vi "FindRobotByRole.vi"(8 "error in (no error)":errorcluster, 9 "role":T1=enum."DefenderArea", 10 "RobotRef":refnum<class "Robot.lvclass">[](array[class]), 11 "Utilities in":refnum<class "Utilities.lvclass">) -> (0 "error out":errorcluster, 2 "Robots":refnum<class "Robot.lvclass">[](array[class]), 3 "Utilities out":refnum<class "Utilities.lvclass">)   [LabVIEW 2023, in "Utilities.lvclass"]
uses:
  Utilities.lvclass
  Robot_class/Robot.lvclass
  Robot_class/roles.ctl
  Robot_class/Robot.lvclass/Robot.ctl
  Robot_class/Read role.vi
panel:
  out "Roles":T1[](array[typedef])
  out "role 2":i32
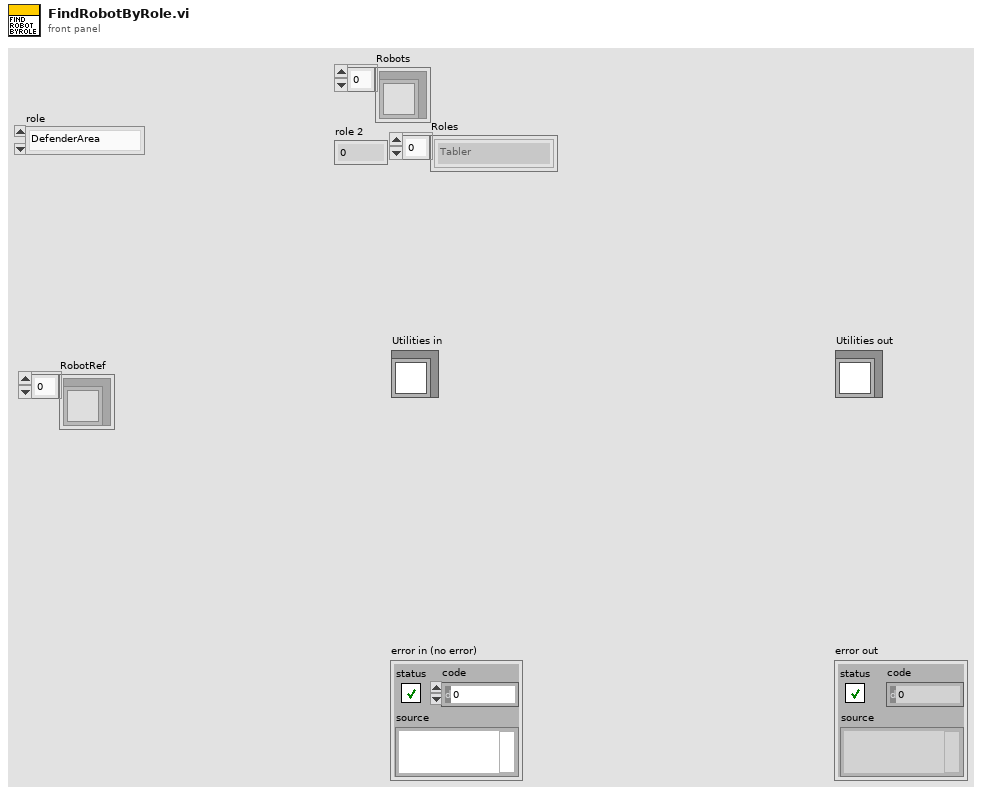
[diagram p1: front panel]
types:
  T1 = typedef "roles.ctl" = enum16{"BallChallengerAttackerVSS", "NormalAttackerVSS", "AttackerAimGoalVSS", "DefenderAreaVSS", "KeeperVSS", "Tabler", "TableFinalizer", "PrepareRollToPassRoller", "PrepareRollToPassReceiver", "SimplePassRoll", "SimplePassRollReceiver", "PenaltyDefense", "PreparePassReceiver 2", "PreparePassReceiver 1", "PassObserver", "Timeout", "Goto", "ZigZag", "None", "BallOutOfField", "DefenderArea", "Duelist", "AttackerStop", "FollowAttacker", "KeeperRole", "KickPenalty", "AttackerAimGoal", "AttackerBlock", "Marker", "Halt", "Shoot", "PassKicker", "PassReceiver", "TestRole", "PenaltyAttacker"}
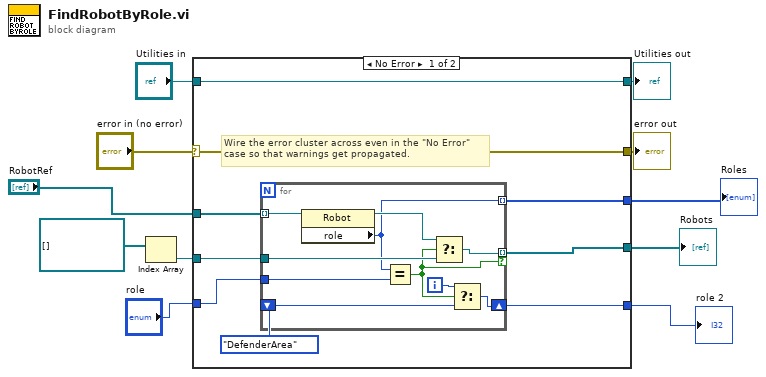
[diagram p0: block diagram]
diagram:
  n1 = Index Array(array=refnum<class "Robot.lvclass">[] []) -> (element=w6:refnum<class "Robot.lvclass">)  [unwired: 1 in]
  n2 = case shown="No Error" "error in (no error)" {
    selector: "error in (no error)" -> [w19 w32]
    tunnel: [w19 w32] -> w10
    tunnel: [w20 w31] -> w8
    tunnel: "Utilities in" -> [w20 w31]
    tunnel: [w18 _] -> w2
    tunnel: w6 -> [w14 _]
    tunnel: "RobotRef" -> [w17 _]
    tunnel: "role" -> [w16 _]
    tunnel: [w13 _] -> w3
    tunnel: [w12 _] -> w1
    frame No Error {
      # "Wire the error cluster across even in the \"No Error\"\ncase so that warnings get propagated."
      n3 = for {
        tunnel: w17 -> [w30] mode=indexing
        tunnel: w16 -> [w29]
        shift-right: [w26] -> w18
        shift-left: roles."DefenderArea" ("role") -> [w25]
        tunnel: w14 -> [w24]
        tunnel: [w23] -> w13 mode=indexing if=w22
        tunnel: [w21] -> w12 mode=indexing
        i -> [w27]
        n4 = property class="Robot"(reference=w30) -> (reference out=w28:refnum<class "Robot.lvclass">, "role"=w21:T1)  [unwired: 1 in, 1 out]
        n5 = Equal?(x=w21, y=w29) -> (x = y?=w22:bool)
        n6 = Select(t=w28, s=w22, f=w24) -> (s? t:f=w23:refnum<class "Robot.lvclass">)
        n7 = Select(t=w27, s=w22, f=w25) -> (s? t:f=w26:i32)
      }
    }
    frame Error {
    }
  }
  "error out" <- w10
  "Utilities out" <- w8
  "Robots" <- w3
  "role 2" <- w2
  "Roles" <- w1
